vi "CORREGGI DATABASE MISURE.vi"() -> ()   [LabVIEW 2019]
uses:
  <vilib>/addons/database/Connection.llb/Conn Execute.vi
  <vilib>/addons/database/Recordset.llb/Rec Fetch Recordset Data (R).vi
  <vilib>/addons/database/_DB Variant To Data/Database Variant To Data.xnode
  <vilib>/addons/database/NI_Database_API.lvlib
panel:
  out "output array":string[][](array[string])
  in  "SQL query":string="select * from Misure"
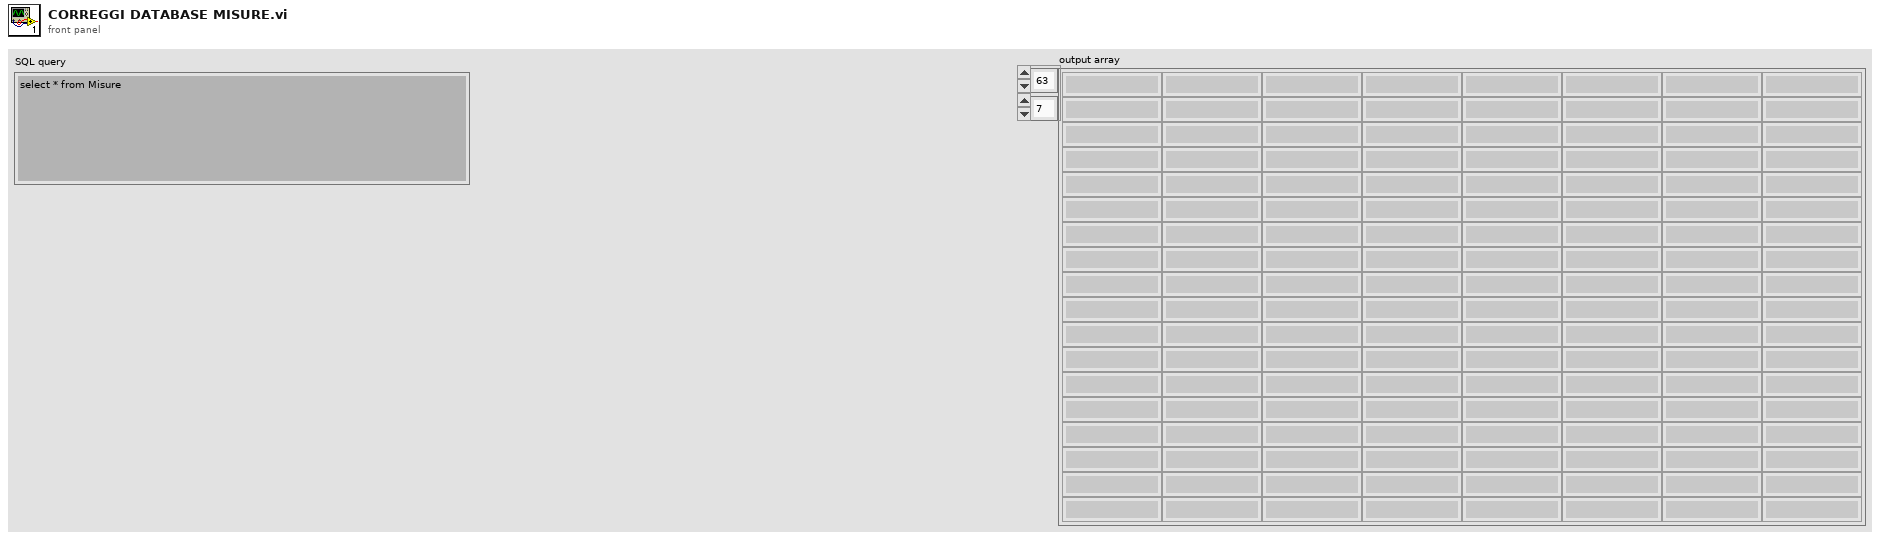
[diagram p1: front panel]
types:
  T1 = typedef "NI_Database_API.lvlib/Conn ObjectReference.ctl" = refnum<k1>
  T2 = typedef "NI_Database_API.lvlib/Rec ObjectReference.ctl" = refnum<k1>
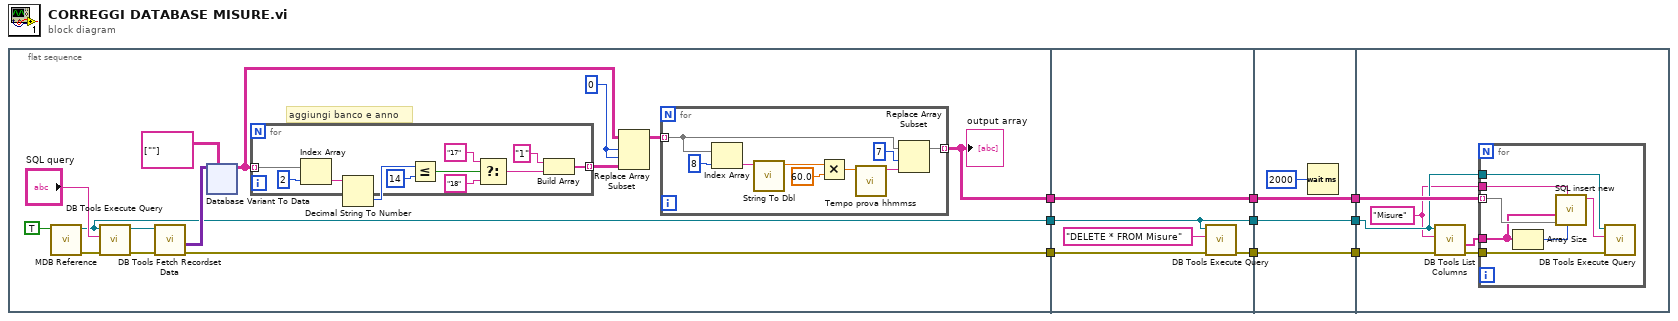
[diagram p0: block diagram]
diagram:
  n1 = flat-sequence {
    tunnel: [w18] -> w9
    tunnel: [w15] -> w8
    tunnel: [w10] -> w7
    tunnel: w9 -> [w92]
    tunnel: w8 -> [w89]
    tunnel: w7 -> [w91]
    tunnel: [w91] -> w6
    tunnel: [w90] -> w4
    tunnel: [w89] -> w2
    tunnel: w6 -> [w96]
    tunnel: [w96] -> w5
    tunnel: w4 -> [w95]
    tunnel: [w95] -> w3
    tunnel: w2 -> [w94]
    tunnel: [w94] -> w1
    tunnel: w5 -> [w101]
    tunnel: w3 -> [w102]
    tunnel: w1 -> [w100]
    frame #0 {
      w14 = 0 ("index (row)")
      # "aggiungi banco e anno"
      n2 = call "MDB Reference.vi"("Collaudi T/motori F"=TRUE ("Collaudi/motori")) -> ("error out"=w16:errorcluster, "Refnum out"=w15:T1)  [unwired: 8 in, 1 out]
      n3 = call-poly <vilib>:"DB Tools Execute Query.vi"("error in (no error)"=w16, "SQL query"="SQL query", "connection reference"=w15) -> ("error out"=w17:errorcluster, "recordset reference"=w22:T2)  [unwired: 5 in]
      n4 = call-poly <vilib>:"DB Tools Fetch Recordset Data.vi"("error in (no error)"=w17, "recordset reference"=w22) -> ("error out"=w18:errorcluster, "recordset data"=w21:variant[][])  [unwired: 3 in, 1 out]
      n5 = xnode "Database Variant To Data"("database variant"=w21, "type"=string[][] [[""]]) -> ("data"=w13:string[][])  [unwired: 1 in, 1 out]
      n6 = for {
        tunnel: w13 -> [w43] mode=indexing
        tunnel: [w33] -> w12 mode=indexing
        n7 = Index Array(array=w43, index=2) -> (element=w41:string)
        n8 = Decimal String To Number(string=w41) -> (number=w40:i32)  [unwired: 2 in, 1 out]
        n9 = Less Or Equal?(x=w40, y=14) -> (x <= y?=w38:bool)
        n10 = Select(t="17", s=w38, f="18") -> (s? t:f=w35:string)
        n11 = Build Array("1" ("element"), w35) -> (w33:string[])
      }
      n12 = Replace Array Subset(array=w13, new element=w12, index (row)=w14, index (col)=w14) -> (w11:string[][])
      n13 = for {
        tunnel: w11 -> [w29] mode=indexing
        tunnel: [w26] -> w10 mode=indexing
        n14 = Index Array(array=w29, index=8) -> (element=w25:string)
        n15 = call "String To Dbl.vi"("String"=w25) -> ("Numeric"=w24:dbl)  [unwired: 10 in]
        n16 = Multiply(x=w24, y=60.0) -> (x*y=w30:dbl)
        n17 = call "Tempo prova hhmmss.vi"("Tempo [s]"=w30) -> ("H:m:s"=w27:string)  [unwired: 10 in]
        n18 = Replace Array Subset(array=w29, new element=w27, index=7) -> (w26:string[])
      }
      "output array" <- w10
    }
    frame #1 {
      n19 = call-poly <vilib>:"DB Tools Execute Query.vi"("error in (no error)"=w92, "SQL query"="DELETE * FROM Misure", "connection reference"=w89) -> ("error out"=w90:errorcluster)  [unwired: 5 in, 1 out]
    }
    frame #2 {
      n20 = Wait (ms)(milliseconds to wait=u32 2000) -> ()  [unwired: 1 out]
    }
    frame #3 {
      w98 = "Misure" ("table")
      n21 = call <vilib>:"DB Tools List Columns.vi"("error in (no error)"=w102, "table"=w98, "connection reference"=w100) -> ("error out"=w97:errorcluster, "columns"=w99:string[])  [unwired: 3 out]
      n22 = for {
        tunnel: w99 -> [w107]
        tunnel: w101 -> [w109] mode=indexing
        tunnel: w98 -> [w108]
        tunnel: w100 -> [w105]
        tunnel: w97 -> [w103]
        n23 = Array Size(array=w107) -> (size(s)=w106:i32)
        n24 = call "SQL insert new .vi"("Numeric 2"=w106, "Nome Tabella"=w108, "ArrayValoriCampi1D"=w109, "ArrayNomiCampi1D"=w107) -> ("output"=w104:string)  [unwired: 7 out]
        n25 = call-poly <vilib>:"DB Tools Execute Query.vi"("error in (no error)"=w103, "SQL query"=w104, "connection reference"=w105) -> ()  [unwired: 5 in, 2 out]
      }
    }
  }
